vi "Solution part 2.vi"() -> ()   [LabVIEW 2020]
panel:
  out "result":i32
  in  "data?":bool
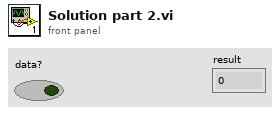
[diagram p1: front panel]
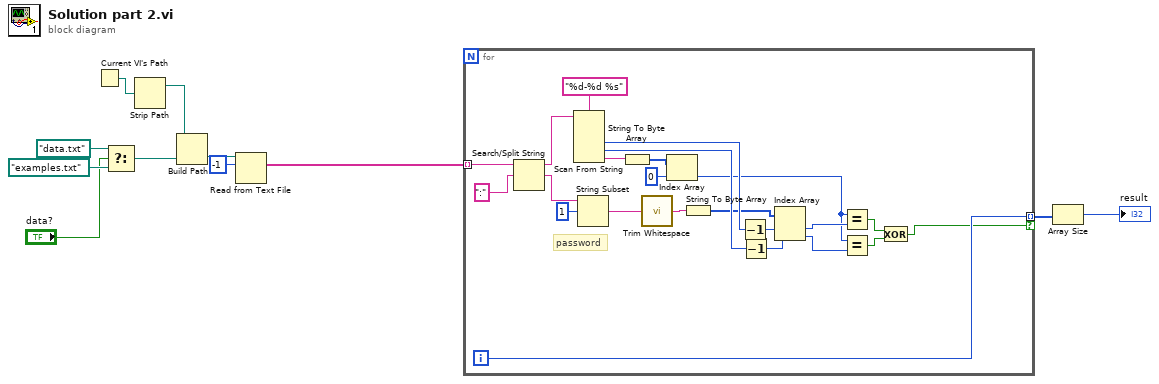
[diagram p0: block diagram]
diagram:
  n1 = Current VI's Path() -> (path=w7:path)
  n2 = Select(t=path "data.txt", s="data?", f=path "examples.txt") -> (s? t:f=w8:path)
  n3 = Strip Path(path=w7) -> (stripped path=w6:path)  [unwired: 1 out]
  n4 = Build Path(base path=w6, name or relative path=w8) -> (appended path=w5:path)
  n5 = Read from Text File(file (use dialog)=w5, count=-1) -> (text=w1:string[])  [unwired: 2 in, 3 out]
  n6 = for {
    tunnel: w1 -> [w34] mode=indexing
    tunnel: [w24] -> w4 mode=indexing if=w12
    i -> [w24]
    # "password"
    n7 = Search/Split String(string=w34, search string/char (-)=":") -> (substring before match=w29:string, match + rest of string=w32:string)  [unwired: 1 in, 1 out]
    n8 = Scan From String(format string="%d-%d %s", input string=w29) -> (output 1=w20:i32, output 2=w19:i32, output 3=w27:string)  [unwired: 5 in, 3 out]
    n9 = String Subset(string=w32, offset (0)=1) -> (substring=w28:string)  [unwired: 1 in]
    n10 = String To Byte Array(string=w27) -> (unsigned byte array=w26:u8[])
    n11 = call <vilib>:"Trim Whitespace.vi"("string"=w28) -> ("trimmed string"=w23:string)  [unwired: 1 in]
    n12 = Index Array(array=w26, index=0) -> (element=w15:u8)
    n13 = String To Byte Array(string=w23) -> (unsigned byte array=w16:u8[])
    n14 = Decrement(x=w20) -> (x-1=w22:i32)
    n15 = Decrement(x=w19) -> (x-1=w21:i32)
    n16 = Index Array(array=w16, index #1=w22, index #2=w21) -> (element #1=w18:u8, element #2=w17:u8)
    n17 = Equal?(x=w15, y=w18) -> (x = y?=w13:bool)
    n18 = Equal?(x=w15, y=w17) -> (x = y?=w14:bool)
    n19 = Exclusive Or(1:w14, 2:w13) -> (0:w12:bool)
  }
  n20 = Array Size(array=w4) -> (size(s)=→"result":i32)
